vi "Frequency Analysis (SubVI).vi"(11 "Filtered Signal":dynamicdata(waveform)) -> (1 "Dynamic Data":dynamicdata(waveform), 2 "Dynamic Data 2":dynamicdata(waveform), 3 "Power Spectrum":dynamicdata(waveform))   [LabVIEW 2021]
uses:
  <vilib>/express/express analysis/Spectral/Block/exnSpectralBlock spectral measurements power poly.vi
  <vilib>/express/express analysis/Spectral/Block/exnSpectralBlock spectral measurements power DDT.vi
  <vilib>/express/express analysis/Spectral/XNode/ExpressSpectralMeasurementsBlockNode.xnode
  <vilib>/Analysis/NI_AALPro.lvlib
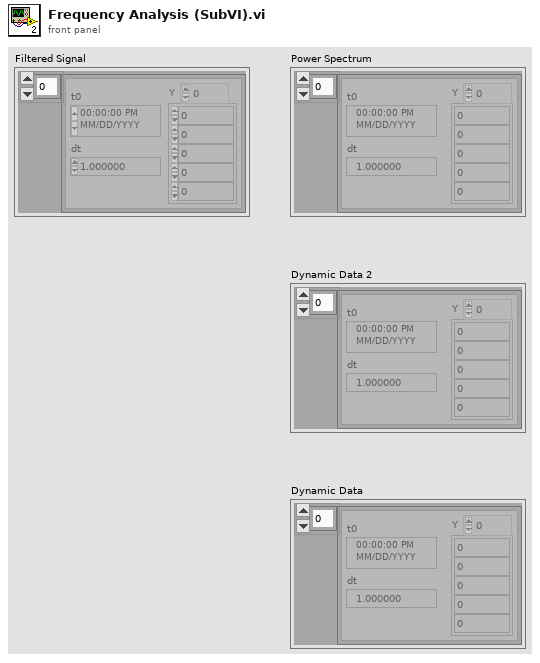
[diagram p1: front panel]
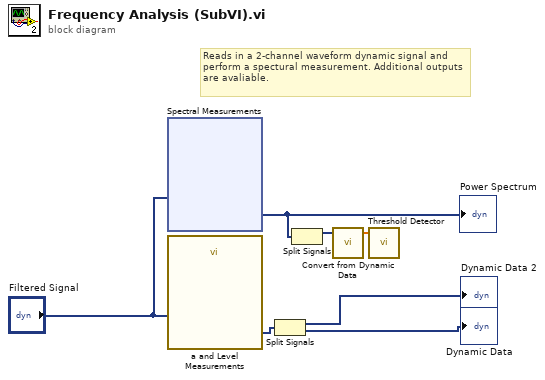
[diagram p0: block diagram]
diagram:
  # "Reads in a 2-channel waveform dynamic signal and perform a spectural measurement. Additional outputs are avaliable."
  n1 = xnode "Spectral Measurements"("Signals"="Filtered Signal") -> ("Power Spectrum"=w4:dynamicdata)  [unwired: 1 in, 1 out]
  "Power Spectrum" <- w4
  n2 = call "a and Level Measurements"("Signals"="Filtered Signal") -> ("Peak to Peak"=w1:dynamicdata)  [unwired: 12 in, 2 out]
  n3 = Split Signals(w1) -> (→"Dynamic Data 2":dynamicdata, →"Dynamic Data":dynamicdata)  [unwired: 2 in]
  n4 = Split Signals(w4) -> (w5:dynamicdata)  [unwired: 2 in, 1 out]
  n5 = call "Convert from Dynamic Data"("Dynamic Data Type"=w5) -> ("Array"=w3:dbl[])  [unwired: 3 in]
  n6 = call <vilib>:"Threshold Detector.vi"("X"=w3) -> ()  [unwired: 2 in, 3 out]
